vi "Replace XML Node from path.vi"(2 "error in":errorcluster, 3 "Data":string="test", 4 "XPath Expression":string="/TestStructure/example/Sample", 5 "XML String":string="<?xml version=\"1.0\" encoding=\"utf-8\"?>\n<TestStructure>\n  <example>\n  <Sample>0</Sample>\n  <Sample2>0</Sample2>\n  </example>\n</TestStructure>") -> (0 "error out":errorcluster, 1 "XML":string)   [LabVIEW 2016]
uses:
  <vilib>/xml/Load XML String.vi
  <vilib>/xml/Close Reference(Node).vi
  <vilib>/regexp/Match Regular Expression.xnode
  <vilib>/xml/NI_XML.lvlib
  <resource>/objmgr/DOMUserDefRef.rc
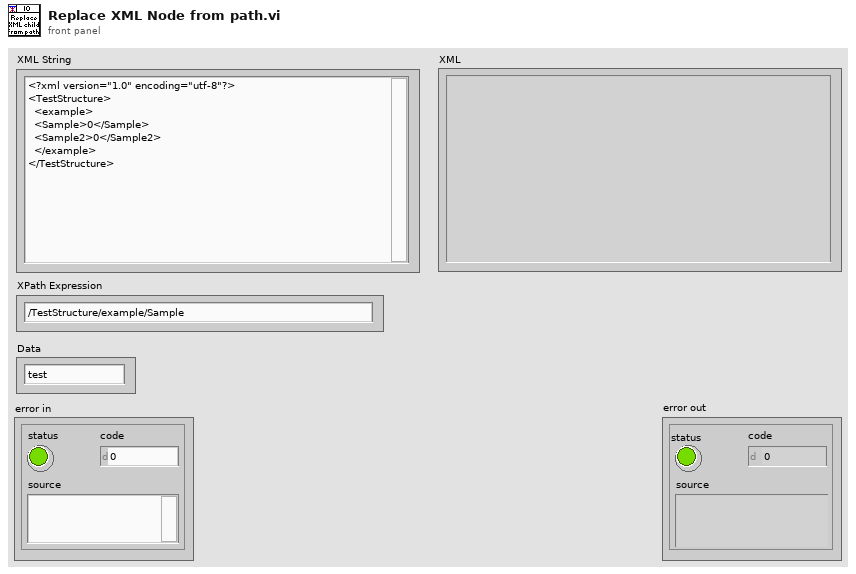
[diagram p1: front panel]
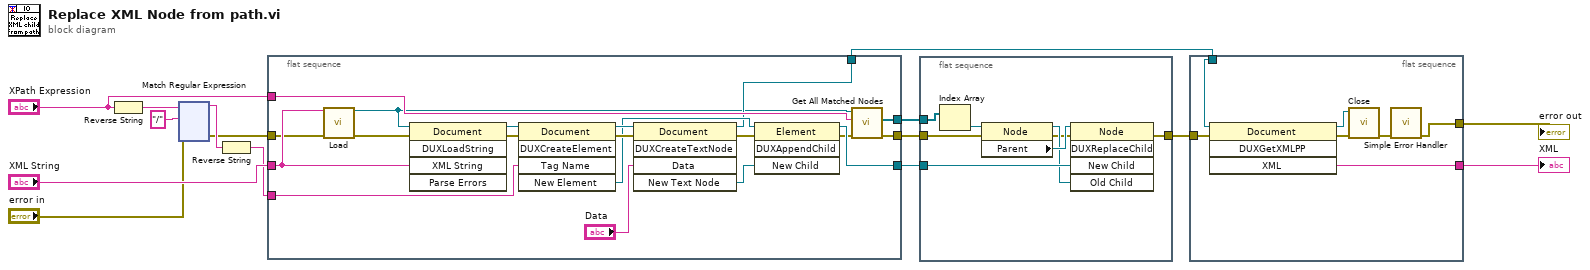
[diagram p0: block diagram]
diagram:
  n1 = Reverse String(1:"XPath Expression") -> (0:w6:string)
  n2 = xnode "Match Regular Expression"("input string"=w6, "regular expression"="/" ("search string/char (-)"), "error in"="error in") -> ("before match"=w7:string, "error out"=w4:errorcluster)  [unwired: 3 in, 3 out]
  n3 = Reverse String(1:w7) -> (0:w5:string)
  n4 = flat-sequence {
    tunnel: [w34] -> w15
    tunnel: [w33] -> w14
    tunnel: "XPath Expression" -> [w32]
    tunnel: "XML String" -> [w31]
    tunnel: w5 -> [w29]
    tunnel: [w23] -> w13
    tunnel: [w22] -> w12
    tunnel: w4 -> [w18]
    frame #0 {
      n5 = call-poly <vilib>:"Load.vi"("XML string"=w31, "error in (no error)"=w18) -> ("DOM document out"=w21:refnum<k20>, "error out"=w17:errorcluster)  [unwired: 11 in, 1 out]
      n6 = invoke class="Document" method="DUXLoadString"(reference=w21, error in=w17, "XML String"=w31) -> (reference out=w30:refnum<k20>, error out=w20:errorcluster)  [unwired: 2 in, 3 out]
      n7 = invoke class="Document" method="DUXCreateElement"(reference=w30, error in=w20, "Tag Name"=w29) -> (reference out=w28:refnum<k20>, error out=w27:errorcluster, "New Element"=w25:refnum<k20>)  [unwired: 2 in, 2 out]
      n8 = invoke class="Document" method="DUXCreateTextNode"(reference=w28, error in=w27, "Data"="Data") -> (reference out=w22:refnum<k20>, error out=w19:errorcluster, "New Text Node"=w24:refnum<k20>)  [unwired: 2 in, 2 out]
      n9 = invoke class="Element" method="DUXAppendChild"(reference=w25, error in=w19, "New Child"=w24) -> (reference out=w23:refnum<k20>, error out=w16:errorcluster)  [unwired: 1 in, 2 out]
      n10 = call <vilib>:"Get All Matched Nodes.vi"("error in (no error)"=w16, "XPath expression"=w32, "node in"=w21) -> ("error out"=w33:errorcluster, "node result array"=w34:refnum<k20>[])  [unwired: 7 out]
    }
  }
  n11 = flat-sequence {
    tunnel: w15 -> [w42]
    tunnel: w14 -> [w37]
    tunnel: w13 -> [w41]
    tunnel: [w35] -> w3
    frame #0 {
      n12 = Index Array(array=w42) -> (element=w38:refnum<k20>)  [unwired: 1 in]
      n13 = property class="Node"(reference=w38, error in=w37) -> (reference out=w39:refnum<k20>, error out=w36:errorcluster, "Parent"=w40:refnum<k20>)
      n14 = invoke class="Node" method="DUXReplaceChild"(reference=w40, error in=w36, "New Child"=w41, "Old Child"=w39) -> (error out=w35:errorcluster)  [unwired: 1 in, 4 out]
    }
  }
  n15 = flat-sequence {
    tunnel: w12 -> [w47]
    tunnel: [w46] -> w11
    tunnel: w3 -> [w45]
    tunnel: [w43] -> w1
    frame #0 {
      n16 = invoke class="Document" method="DUXGetXMLPP"(reference=w47, error in=w45) -> (reference out=w48:refnum<k20>, error out=w44:errorcluster, "XML"=w46:string)  [unwired: 2 in, 1 out]
      n17 = call-poly <vilib>:"Close.vi"("error in (no error)"=w44, "node"=w48) -> ("error out"=w49:errorcluster)  [unwired: 7 out]
      n18 = call <vilib>:"Simple Error Handler.vi"("error in (no error)"=w49) -> ("error out"=w43:errorcluster)  [unwired: 1 in, 7 out]
    }
  }
  "XML" <- w11
  "error out" <- w1
